vi "response.Has ID.vi"(8 "error in (no error)":errorcluster, 11 "Response in":refnum<class "Response.lvclass">) -> (0 "error out":errorcluster, 2 "has id?":bool, 3 "Response out":refnum<class "Response.lvclass">)   [LabVIEW 2016, in "Response.lvclass"]
uses:
  Response.lvclass
  <vilib>/NI/JSON Support for LabVIEW/JSON Types.ctl
  Response.lvclass/Response.ctl
  id/id.Get ID Type.vi
  id/id.lvclass
  <vilib>/NI/JSON Support for LabVIEW/LVJSON.lvlib
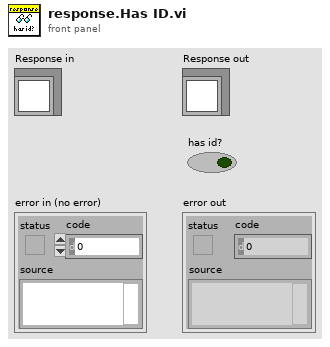
[diagram p1: front panel]
types:
  T1 = typedef "LVJSON.lvlib/JSON Types.ctl" = enum16{"String", "Numeric", "Boolean", "NULL", "Object", "Array"}
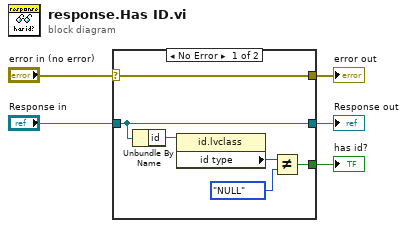
[diagram p0: block diagram]
diagram:
  n1 = case shown="No Error" "error in (no error)" {
    selector: "error in (no error)" -> [w11 w13]
    tunnel: [w11 w13] -> w4
    tunnel: [w10 w12] -> w2
    tunnel: "Response in" -> [w10 w12]
    tunnel: [w9 _] -> w1
    frame No Error {
      n2 = Unbundle By Name(w10) -> ("id"=w8:refnum<class "id.lvclass">)
      n3 = property class="id.lvclass"(reference=w8) -> ("id type"=w7:T1)  [unwired: 1 in, 2 out]
      n4 = Not Equal?(x=w7, y=JSON_Types."NULL") -> (x != y?=w9:bool)
    }
    frame Error {
    }
  }
  "error out" <- w4
  "Response out" <- w2
  "has id?" <- w1
